vi "rpm converter.vi"(9 "y":dbl=255.0) -> (1 "x-y":dbl format="%#.3g")   [LabVIEW 2021]
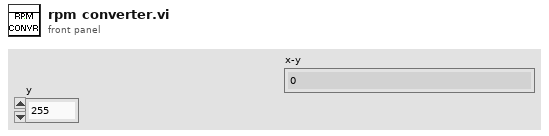
[diagram p1: front panel]
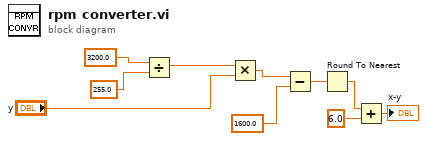
[diagram p0: block diagram]
diagram:
  n1 = Divide(x=3200.0, y=255.0) -> (x/y=w8:dbl)
  n2 = Multiply(x=w8, y="y") -> (x*y=w6:dbl)
  n3 = Subtract(x=w6, y=1600.0) -> (x-y=w4:dbl)
  n4 = Round To Nearest(number=w4) -> (nearest integer value=w3:dbl)
  n5 = Add(x=w3, y=6.0) -> (x+y=→"x-y":dbl)
